vi "CTRE_CANTalonSRX_ChangeMode.vi"(6 "Master Device Number":u8, 8 "error in (no error)":errorcluster, 9 "Output":dbl, 10 "Talon SRX Control Mode":T1, 11 "CAN Talon SRX Ref":T2={"DeviceStatus"={"status"=FALSE, "code"=0, "source"=""}, "Type"=enum."PWM", "PWM"={"PWM Channel"=enum."PWM 1", "DeadBand"={"Name"="", "maxPositivePwm"=0, "minPositivePwm"=0, "centerPwm"=0, "maxNegativePwm"=0, "minNegativePwm"=0, "angularRange"=0}}, "CAN"={"Device Number"=0, "SetOutput VI Ref"=variant(enum8{"Percent VBus", "Current", "Speed", "Position", "Voltage"} enum."Percent VBus"), "GetOutput VI Ref"=variant(refnum<k1> refnum), "Enable VI Ref"=variant(dbl 12.0), "Disable VI Ref"=variant(enum8{"Percent VBus", "Speed", "Position", "Slave", "Unchanged / Invalid", "Voltage Compensation", "Current", "Motion Profile"} enum."Percent VBus"), "Data"=variant}, "Invert"=FALSE}) -> (0 "error out":errorcluster, 3 "CAN Talon SRX Ref":T2={"DeviceStatus"={"status"=FALSE, "code"=0, "source"=""}, "Type"=enum."PWM", "PWM"={"PWM Channel"=enum."PWM 1", "DeadBand"={"Name"="", "maxPositivePwm"=0, "minPositivePwm"=0, "centerPwm"=0, "maxNegativePwm"=0, "minNegativePwm"=0, "angularRange"=0}}, "CAN"={"Device Number"=0, "SetOutput VI Ref"=variant(enum8{"Percent VBus", "Current", "Speed", "Position", "Voltage"} enum."Percent VBus"), "GetOutput VI Ref"=variant(refnum<k1> refnum), "Enable VI Ref"=variant(dbl 12.0), "Disable VI Ref"=variant(enum8{"Percent VBus", "Speed", "Position", "Slave", "Unchanged / Invalid", "Voltage Compensation", "Current", "Motion Profile"} enum."Percent VBus"), "Data"=variant}, "Invert"=FALSE})   [LabVIEW 2016]
doc: "Changes the Control Mode of the Talon SRX.\n\nYou must also set the output value when changing the mode.\n\n<B>Master Device Number</B> is the CAN bus device ID of the master controller and must be set if placing the current Talon SRX into \"Slave\" mode."
uses:
  <vilib>/Rock Robotics/WPI/MotorControl/WPI_MotorControlDeviceRef.ctl
  <vilib>/Rock Robotics/WPI/MotorControl/WPI_MotorControlType.ctl
  <vilib>/Rock Robotics/SystemInterfaces/DIO/FPGA_DIOPWMChannel.ctl
  <vilib>/Rock Robotics/WPI/PWM/WPI_PWMDeadband.ctl
  <vilib>/Rock Robotics/WPI/ThirdParty/CanMotor/CTRLib-LV-TalonSRX/CTRE_CANTalonSRX_ControlMode.ctl
  <vilib>/Rock Robotics/WPI/ThirdParty/CanMotor/CTRLib-LV-TalonSRX/TalonSRXDevRefData.ctl
  <vilib>/Rock Robotics/WPI/ThirdParty/CanMotor/CTRLib-LV-TalonSRX/CTRE_CANTalonSRX_UsageTypes.ctl
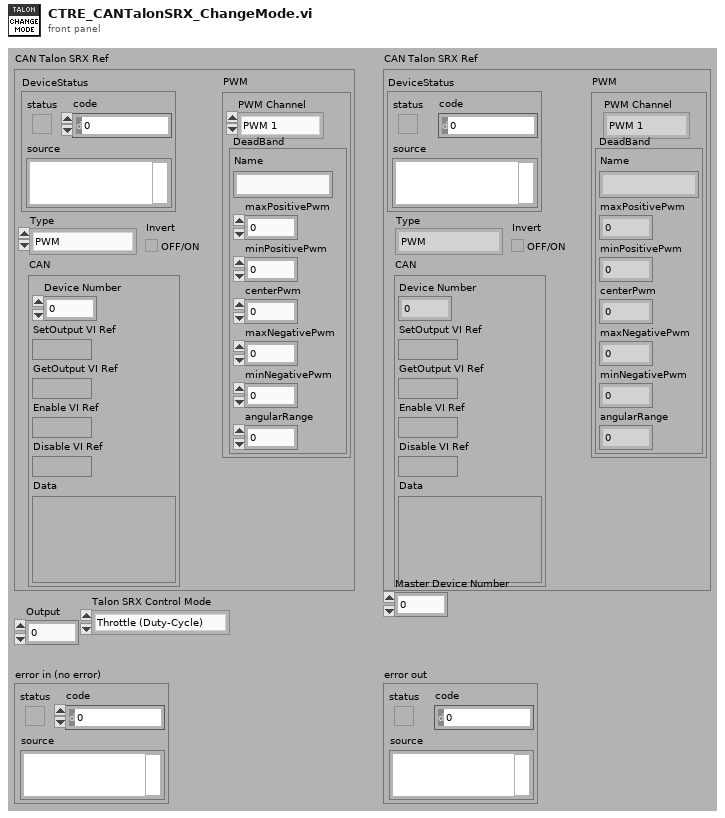
[diagram p1: front panel]
types:
  T1 = typedef "CTRE_CANTalonSRX_ControlMode.ctl" = enum16{"Throttle (Duty-Cycle)", "Position Closed-Loop", "Velocity Closed-Loop", "Current Closed-Loop", "Voltage Compensation", "Slave Follower", "Motion Profile", "Motion Magic"}
  T2 = typedef "WPI_MotorControlDeviceRef.ctl" = cluster{"DeviceStatus":errorcluster, "Type":T3, "PWM":cluster{"PWM Channel":T4, "DeadBand":T5}, "CAN":cluster{"Device Number":u8, "SetOutput VI Ref":variant, "GetOutput VI Ref":variant, "Enable VI Ref":variant, "Disable VI Ref":variant, "Data":variant}, "Invert":bool}
  T3 = typedef "WPI_MotorControlType.ctl" = enum16{"PWM", "CAN"}
  T4 = typedef "FPGA_DIOPWMChannel.ctl" = enum8{"PWM 0", "PWM 1", "PWM 2", "PWM 3", "PWM 4", "PWM 5", "PWM 6", "PWM 7", "PWM 8", "PWM 9", "PWM MXP 0", "PWM MXP 1", "PWM MXP 2", "PWM MXP 3", "PWM MXP 4", "PWM MXP 5", "PWM MXP 6", "PWM MXP 7", "PWM MXP 8", "PWM MXP 9", "Invalid"}
  T5 = typedef "WPI_PWMDeadband.ctl" = cluster{"Name":string, "maxPositivePwm":i32, "minPositivePwm":i32, "centerPwm":i32, "maxNegativePwm":i32, "minNegativePwm":i32, "angularRange":u16}
  T6 = typedef "TalonSRXDevRefData.ctl" = cluster{"Library":path, "handle":u64, "Talon SRX Mode":T1, "UsageFrame":u32, "RefNumName":string}
  T7 = typedef "CTRE_CANTalonSRX_UsageTypes.ctl" = u32
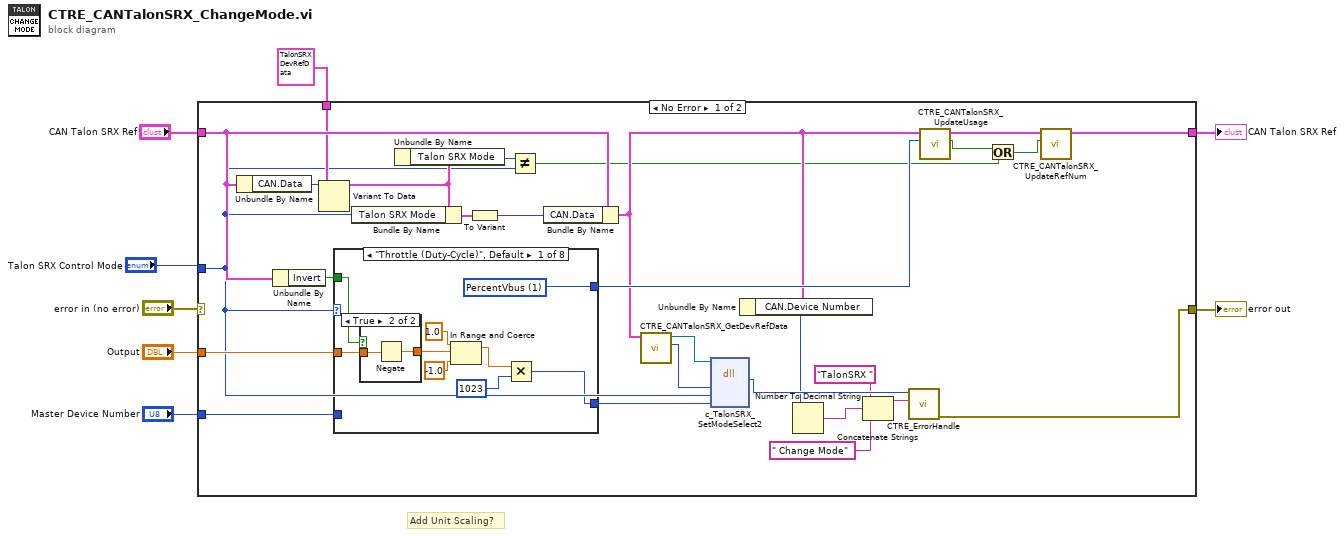
[diagram p0: block diagram]
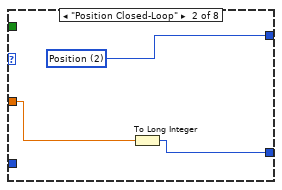
[diagram p3: hidden frame]
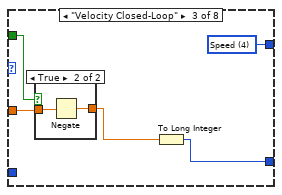
[diagram p4: hidden frame]
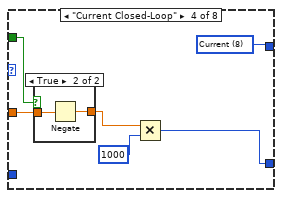
[diagram p6: hidden frame]
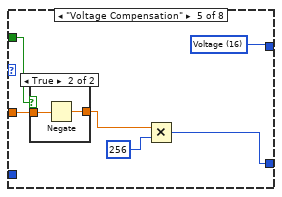
[diagram p8: hidden frame]
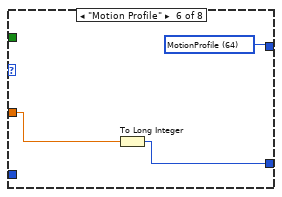
[diagram p10: hidden frame]
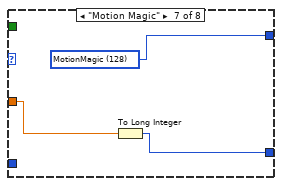
[diagram p11: hidden frame]
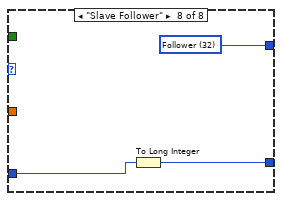
[diagram p12: hidden frame]
diagram:
  # "Add Unit Scaling?"
  n1 = case shown="No Error" "error in (no error)" {
    selector: "error in (no error)" -> [_ w88]
    tunnel: [w23 w88] -> w8
    tunnel: [w15 w87] -> w6
    tunnel: "CAN Talon SRX Ref" -> [w21 w87]
    tunnel: "Talon SRX Control Mode" -> [w10 _]
    tunnel: "Output" -> [w31 _]
    tunnel: "Master Device Number" -> [w35 _]
    tunnel: T6 {"Library"=path "", "handle"=0, "Talon SRX Mode"=enum."Throttle (Duty-Cycle)", "UsageFrame"=0, "RefNumName"=""} ("Cluster") -> [w20 _]
    frame No Error {
      n2 = Unbundle By Name(w21) -> ("CAN.Data"=w17:variant)
      n3 = Unbundle By Name(w21) -> ("Invert"=w30:bool)
      n4 = Variant To Data(type=w20, Variant=w17) -> (data=w12:T6)  [unwired: 1 in, 1 out]
      n5 = case shown="\"Throttle (Duty-Cycle)\", Default" w10 {
        tunnel: [w45 w51 w56 w65 w74 w80 w83 w86] -> w36
        tunnel: w35 -> [_ _ _ _ _ _ _ w85]
        tunnel: [w37 w49 w52 w60 w69 w78 w81 w84] -> w34
        tunnel: w31 -> [w43 w50 w55 w64 w73 w79 w82 _]
        tunnel: w30 -> [w44 _ w54 w63 w72 _ _ _]
        frame "Throttle (Duty-Cycle)", Default {
          w45 = T7 1 items=["Default"=0, "PercentVbus"=1, "Position"=2, "Speed"=4, "Current"=8, "Voltage"=16, "Follower"=32, "MotionProfile"=64, "MotionMagic"=128, "VRampRate"=4194304, "CurrentLimit"=8388608, "ZeroSensorI"=16777216, "ZeroSensorF"=33554432, "ZeroSensorR"=67108864, "ForwardLimitSwitch"=134217728, "ReverseLimitSwitch"=268435456, "ForwardSoftLimit"=536870912, "ReverseSoftLimit"=1073741824, "MultiProfile"=2147483648]
          n6 = case shown="True" w44 {
            tunnel: w43 -> [w46 w48]
            tunnel: [w46 w47] -> w42
            frame False {
            }
            frame True {
              n7 = Negate(x=w48) -> (-x=w47:dbl)
            }
          }
          n8 = In Range and Coerce(upper limit=1.0, x=w42, lower limit=-1.0) -> (coerced(x)=w39:dbl)  [unwired: 1 out]
          n9 = Multiply(x=w39, y=u32 1023) -> (x*y=w37:i32)
        }
        frame "Position Closed-Loop" {
          w51 = T7 2 items=["Default"=0, "PercentVbus"=1, "Position"=2, "Speed"=4, "Current"=8, "Voltage"=16, "Follower"=32, "MotionProfile"=64, "MotionMagic"=128, "VRampRate"=4194304, "CurrentLimit"=8388608, "ZeroSensorI"=16777216, "ZeroSensorF"=33554432, "ZeroSensorR"=67108864, "ForwardLimitSwitch"=134217728, "ReverseLimitSwitch"=268435456, "ForwardSoftLimit"=536870912, "ReverseSoftLimit"=1073741824, "MultiProfile"=2147483648]
          n10 = To Long Integer(number=w50) -> (32bit integer=w49:i32)
        }
        frame "Velocity Closed-Loop" {
          w56 = T7 4 items=["Default"=0, "PercentVbus"=1, "Position"=2, "Speed"=4, "Current"=8, "Voltage"=16, "Follower"=32, "MotionProfile"=64, "MotionMagic"=128, "VRampRate"=4194304, "CurrentLimit"=8388608, "ZeroSensorI"=16777216, "ZeroSensorF"=33554432, "ZeroSensorR"=67108864, "ForwardLimitSwitch"=134217728, "ReverseLimitSwitch"=268435456, "ForwardSoftLimit"=536870912, "ReverseSoftLimit"=1073741824, "MultiProfile"=2147483648]
          n11 = case shown="True" w54 {
            tunnel: w55 -> [w57 w59]
            tunnel: [w57 w58] -> w53
            frame False {
            }
            frame True {
              n12 = Negate(x=w59) -> (-x=w58:dbl)
            }
          }
          n13 = To Long Integer(number=w53) -> (32bit integer=w52:i32)
        }
        frame "Current Closed-Loop" {
          w65 = T7 8 items=["Default"=0, "PercentVbus"=1, "Position"=2, "Speed"=4, "Current"=8, "Voltage"=16, "Follower"=32, "MotionProfile"=64, "MotionMagic"=128, "VRampRate"=4194304, "CurrentLimit"=8388608, "ZeroSensorI"=16777216, "ZeroSensorF"=33554432, "ZeroSensorR"=67108864, "ForwardLimitSwitch"=134217728, "ReverseLimitSwitch"=268435456, "ForwardSoftLimit"=536870912, "ReverseSoftLimit"=1073741824, "MultiProfile"=2147483648]
          n14 = case shown="True" w63 {
            tunnel: w64 -> [w66 w68]
            tunnel: [w66 w67] -> w62
            frame False {
            }
            frame True {
              n15 = Negate(x=w68) -> (-x=w67:dbl)
            }
          }
          n16 = Multiply(x=w62, y=u32 1000) -> (x*y=w60:i32)
        }
        frame "Voltage Compensation" {
          w74 = T7 16 items=["Default"=0, "PercentVbus"=1, "Position"=2, "Speed"=4, "Current"=8, "Voltage"=16, "Follower"=32, "MotionProfile"=64, "MotionMagic"=128, "VRampRate"=4194304, "CurrentLimit"=8388608, "ZeroSensorI"=16777216, "ZeroSensorF"=33554432, "ZeroSensorR"=67108864, "ForwardLimitSwitch"=134217728, "ReverseLimitSwitch"=268435456, "ForwardSoftLimit"=536870912, "ReverseSoftLimit"=1073741824, "MultiProfile"=2147483648]
          n17 = case shown="True" w72 {
            tunnel: w73 -> [w75 w77]
            tunnel: [w75 w76] -> w70
            frame False {
            }
            frame True {
              n18 = Negate(x=w77) -> (-x=w76:dbl)
            }
          }
          n19 = Multiply(x=w70, y=u32 256) -> (x*y=w69:i32)
        }
        frame "Motion Profile" {
          w80 = T7 64 items=["Default"=0, "PercentVbus"=1, "Position"=2, "Speed"=4, "Current"=8, "Voltage"=16, "Follower"=32, "MotionProfile"=64, "MotionMagic"=128, "VRampRate"=4194304, "CurrentLimit"=8388608, "ZeroSensorI"=16777216, "ZeroSensorF"=33554432, "ZeroSensorR"=67108864, "ForwardLimitSwitch"=134217728, "ReverseLimitSwitch"=268435456, "ForwardSoftLimit"=536870912, "ReverseSoftLimit"=1073741824, "MultiProfile"=2147483648]
          n20 = To Long Integer(number=w79) -> (32bit integer=w78:i32)
        }
        frame "Motion Magic" {
          w83 = T7 128 items=["Default"=0, "PercentVbus"=1, "Position"=2, "Speed"=4, "Current"=8, "Voltage"=16, "Follower"=32, "MotionProfile"=64, "MotionMagic"=128, "VRampRate"=4194304, "CurrentLimit"=8388608, "ZeroSensorI"=16777216, "ZeroSensorF"=33554432, "ZeroSensorR"=67108864, "ForwardLimitSwitch"=134217728, "ReverseLimitSwitch"=268435456, "ForwardSoftLimit"=536870912, "ReverseSoftLimit"=1073741824, "MultiProfile"=2147483648]
          n21 = To Long Integer(number=w82) -> (32bit integer=w81:i32)
        }
        frame "Slave Follower" {
          w86 = T7 32 items=["Default"=0, "PercentVbus"=1, "Position"=2, "Speed"=4, "Current"=8, "Voltage"=16, "Follower"=32, "MotionProfile"=64, "MotionMagic"=128, "VRampRate"=4194304, "CurrentLimit"=8388608, "ZeroSensorI"=16777216, "ZeroSensorF"=33554432, "ZeroSensorR"=67108864, "ForwardLimitSwitch"=134217728, "ReverseLimitSwitch"=268435456, "ForwardSoftLimit"=536870912, "ReverseSoftLimit"=1073741824, "MultiProfile"=2147483648]
          n22 = To Long Integer(number=w85) -> (32bit integer=w84:i32)
        }
      }
      n23 = Bundle By Name(cluster=w12, "Talon SRX Mode"=w10) -> (w18:T6)
      n24 = Unbundle By Name(w12) -> ("Talon SRX Mode"=w11:T1)
      n25 = To Variant(anything=w18) -> (Variant=w19:variant)
      n26 = Not Equal?(x=w11, y=w10) -> (x != y?=w9:bool)
      n27 = Bundle By Name(cluster=w21, "CAN.Data"=w19) -> (w22:T2)
      n28 = call <vilib>:"CTRE_CANTalonSRX_GetDevRefData.vi"("MotorControlDevRef"=w22) -> ("handle"=w33:u64, "Library"=w32:path)  [unwired: 6 in, 3 out]
      n29 = dll-call lib="?" fn="c_TalonSRX_SetModeSelect2"(path in=w32, "handle"=w33, "modeSelect"=w10, "demand"=w34) -> ("return type"=w29:i32)  [unwired: 5 in, 2 out]
      n30 = Unbundle By Name(w22) -> ("CAN.Device Number"=w25:u8)
      n31 = Number To Decimal String(number=w25) -> (decimal integer string=w26:string)  [unwired: 1 in]
      n32 = Concatenate Strings("TalonSRX " ("string"), w26, " Change Mode" ("string")) -> (w28:string)
      n33 = call <vilib>:"CTRE_ErrorHandle.vi"("origin"=w28, "code"=w29) -> ("error out"=w23:errorcluster)  [unwired: 9 in]
      n34 = call <vilib>:"CTRE_CANTalonSRX_UpdateUsage.vi"("Usage"=w36, "CAN Talon SRX Ref"=w22) -> ("Update"=w14:bool, "CAN Talon SRX"=w16:T2)  [unwired: 8 in]
      n35 = Or(x=w14, y=w9) -> (x .or. y?=w13:bool)
      n36 = call <vilib>:"CTRE_CANTalonSRX_UpdateRefNum.vi"("Update"=w13, "CAN Talon SRX Ref"=w16) -> ("CAN Talon SRX Ref"=w15:T2)  [unwired: 9 in]
    }
    frame Error {
    }
  }
  "CAN Talon SRX Ref" <- w6
  "error out" <- w8
